vi "Entry.vi"(8 "error in (no error)":errorcluster, 11 "New State":refnum<class "Do Nothing.lvclass">) -> (0 "error out":errorcluster, 3 "State out":refnum<class "Do Nothing.lvclass">)   [LabVIEW 2013, in "Receiver.lvlib" / "Receive Commands Using State Actors.lvlib" / "Do Nothing.lvlib" / "Do Nothing.lvclass"]
doc: "This is an abstract method. Override this method to define the behavior when you enter the state."
uses:
  Do Nothing.lvclass
  Receiver Command.lvclass
  <vilib>/ActorFramework/Actor/Actor.lvclass/Actor.ctl
  <vilib>/ActorFramework/Message Enqueuer/Message Enqueuer.lvclass/Message Enqueuer.ctl
  <vilib>/ActorFramework/Message Enqueuer/Init from Existing Queue.vi
  <vilib>/ActorFramework/Message Enqueuer/Enqueue.vi
  <vilib>/ActorFramework/Message Priority Queue/Priority Enqueue.vi
  <vilib>/ActorFramework/Message Enqueuer/Message Enqueuer.lvclass
  Command State Actor Messages/Go To Completing Msg/Go To Completing Msg.lvclass
  <vilib>/ActorFramework/Actor/Actor.lvclass
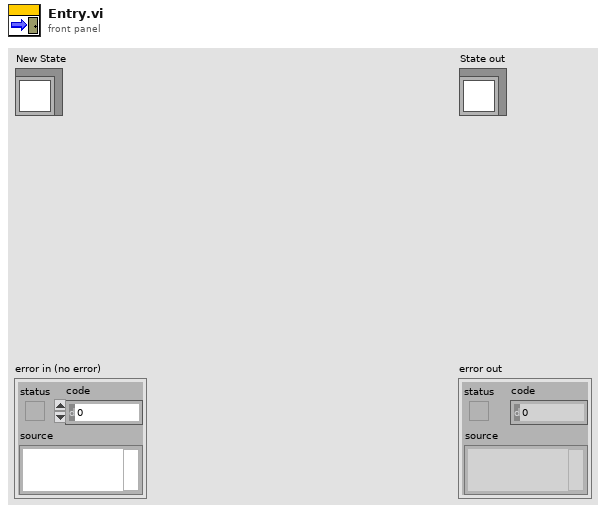
[diagram p1: front panel]
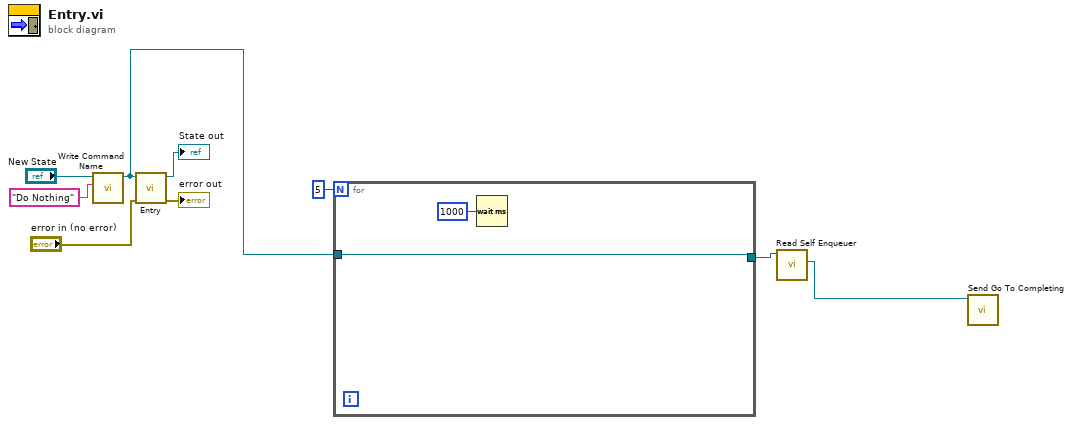
[diagram p0: block diagram]
diagram:
  n1 = call-dynamic "Write Command Name.vi"("Name"="Do Nothing", "Command in"="New State") -> ("Command out"=w2:refnum<class "Do Nothing.lvclass">)  [unwired: 8 in, 1 out]
  n2 = call-parent "Entry.vi"("error in (no error)"="error in (no error)", "New State"=w2) -> ("error out"=→"error out":errorcluster, "State out"=→"State out":refnum<class "Do Nothing.lvclass">)  [unwired: 8 in]
  n3 = for {
    N: 5 -> [_]
    tunnel: [w10] -> w1
    tunnel: w2 -> [w10]
    n4 = Wait (ms)(milliseconds to wait=u32 1000) -> ()  [unwired: 1 out]
  }
  n5 = call <vilib>:"Read Self Enqueuer.vi"("Actor"=w1) -> ("Self Enqueuer"=w4:refnum<class "Message Enqueuer.lvclass">)  [unwired: 10 in]
  n6 = call "Send Go To Completing.vi"("Message Enqueuer"=w4) -> ()  [unwired: 9 in, 2 out]
